vi "Check First Character Type.vi"(1 "Type":u16(ring) items=["Digit, Period or -", "\"", "Character", "Space or Comma"], 2 "Character":string) -> (0 "True/False":bool)   [LabVIEW 2016]
doc: "This VI tests whether a character is of a certain type. It is very useful for parsing."
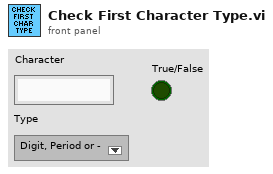
[diagram p1: front panel]
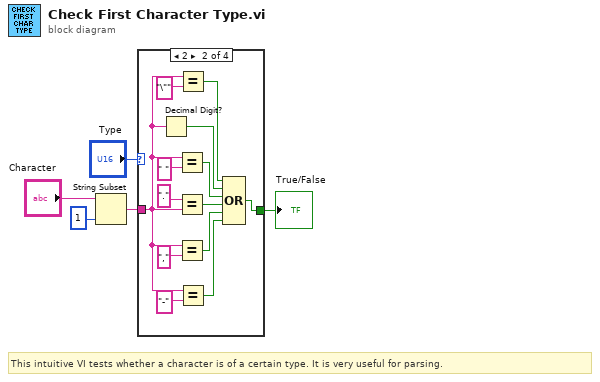
[diagram p0: block diagram]
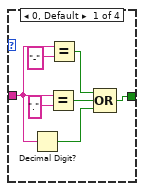
[diagram p2: hidden frame]
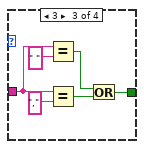
[diagram p3: hidden frame]
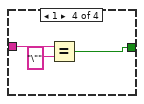
[diagram p4: hidden frame]
diagram:
  # "This intuitive VI tests whether a character is of a certain type. It is very useful for parsing."
  n1 = String Subset(string="Character", length (rest)=1 ("length (rest)")) -> (substring=w2:string)  [unwired: 1 in]
  n2 = case shown="2" "Type" {
    tunnel: w2 -> [w11 w13 w27 w34]
    tunnel: [w6 w24 w31 w32] -> w1
    frame 0, Default {
      n3 = Decimal Digit?(1:w11) -> (0:w7:bool)
      n4 = Equal?(x=w11, y=".") -> (x = y?=w8:bool)
      n5 = Equal?(x=w11, y="-") -> (x = y?=w9:bool)
      n6 = Compound Arithmetic op=OR(w9, w8, w7) -> (w6:bool)
    }
    frame 2 {
      n7 = Decimal Digit?(1:w13) -> (0:w22:bool)
      n8 = Equal?(x=w13, y=" ") -> (x = y?=w18:bool)
      n9 = Equal?(x="." ("y"), y=w13) -> (x = y?=w17:bool)
      n10 = Equal?(x=w13, y=",") -> (x = y?=w16:bool)
      n11 = Equal?(x=w13, y="\"") -> (x = y?=w23:bool)
      n12 = Equal?(x=w13, y="-") -> (x = y?=w14:bool)
      n13 = Compound Arithmetic op=OR(w23, w22, w18, w17, w16, w14) -> (w24:bool)
    }
    frame 3 {
      n14 = Equal?(x=w27, y=" ") -> (x = y?=w30:bool)
      n15 = Equal?(x=w27, y=",") -> (x = y?=w29:bool)
      n16 = Or(x=w30, y=w29) -> (x .or. y?=w31:bool)
    }
    frame 1 {
      n17 = Equal?(x=w34, y="\"") -> (x = y?=w32:bool)
    }
  }
  "True/False" <- w1
